vi "Close.vi"(8 "error in (no error)":errorcluster, 11 "TcpReader in":refnum<class "TcpReader.lvclass">) -> (0 "error out":errorcluster, 3 "TcpReader out":refnum<class "TcpReader.lvclass">)   [LabVIEW 2013, in "TcpReader.lvclass"]
doc: "Closes all open references and reserved resources for the reader"
uses:
  TcpReader.lvclass
  StringReader/StringReader.lvclass
  TcpReader.lvclass/TcpReader.ctl
  Interface/TCP/TCP/TCP.lvclass
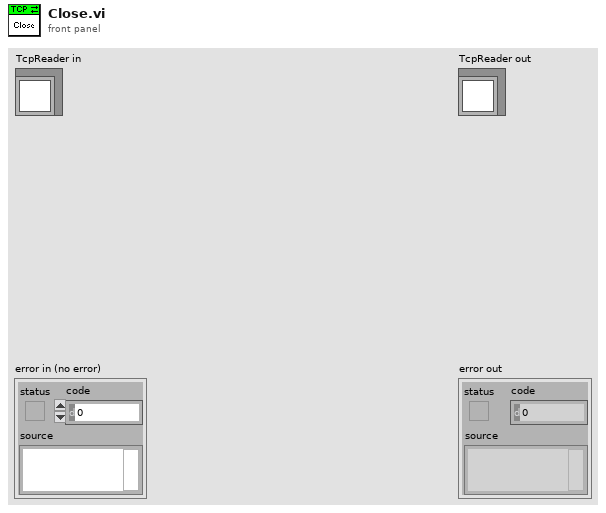
[diagram p1: front panel]
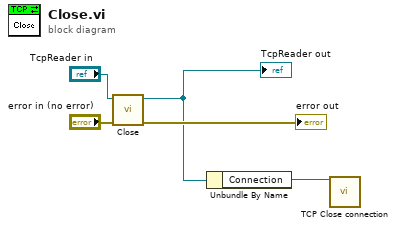
[diagram p0: block diagram]
diagram:
  n1 = call-parent "Close.vi"("error in (no error)"="error in (no error)", "StringReader in"="TcpReader in") -> ("error out"=→"error out":errorcluster, "StringReader out"=w2:refnum<class "TcpReader.lvclass">)  [unwired: 8 in]
  "TcpReader out" <- w2
  n2 = Unbundle By Name(w2) -> ("Connection"=w1:refnum<class "TCP.lvclass">)
  n3 = call-dynamic "TCP Close connection.vi"("TCP in"=w1) -> ()  [unwired: 9 in, 2 out]
